vi "DrawAntennas.vi"(8 "Coords":u32[][](array[numeric]), 10 "New Image":T1, 11 "In Image":T1) -> (3 "Out Image":T1)   [LabVIEW 2024]
uses:
  <vilib>/vision/Image Controls.llb/IMAQ Image.ctl
  <vilib>/vision/NI_Vision_Development_Module.lvlib
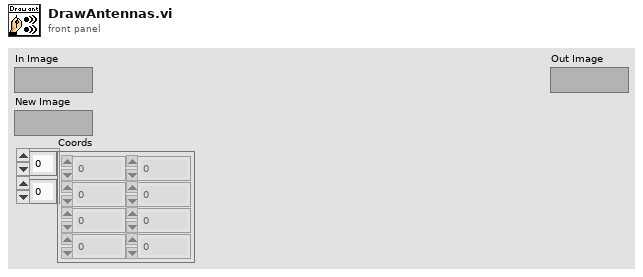
[diagram p1: front panel]
types:
  T1 = typedef "IMAQ Image.ctl" = refnum<image>
  T2 = cluster{"Desired Font (Application)":enum16{"User-specified Font", "Application Font", "System Font", "Dialog Font"}, "[User-specified Font]":cluster{"Font Name":string, "Size":i16, "Strikeout?":bool, "Italic?":bool, "Underline?":bool, "Outline?":bool, "Shadow?":bool, "Bold?":bool, "Rotation Angle":dbl}, "Horizontal Alignment":i16, "Vertical Alignment":i16}
  T3 = cluster{"Red or Hue value":u8, "Green or Sat value":u8, "Blue or Luma or Val or Inten value":u8}
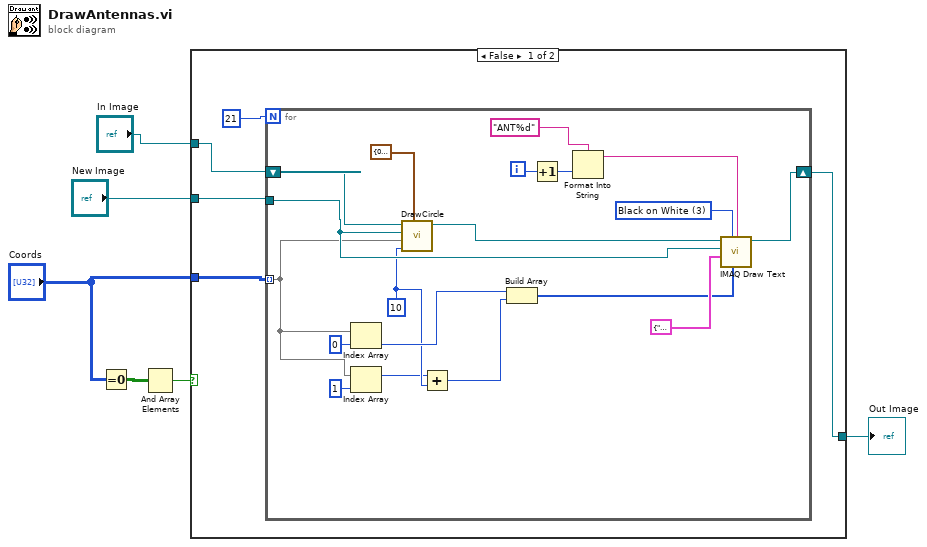
[diagram p0: block diagram]
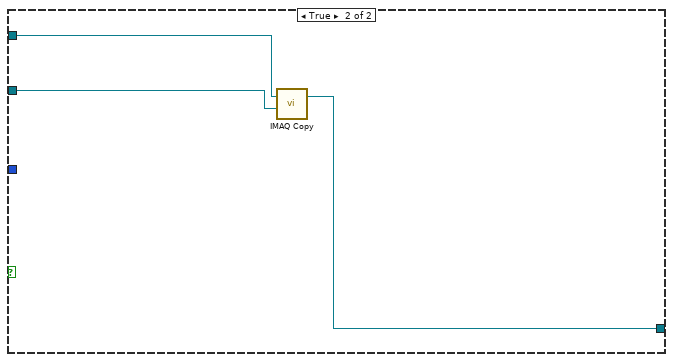
[diagram p2: hidden frame]
diagram:
  n1 = Equal To 0?(x="Coords") -> (x = 0?=w2:bool[][])
  n2 = And Array Elements(Boolean array=w2) -> (logical AND=w1:bool)
  n3 = case shown="False" w1 {
    tunnel: [w10 w31] -> w6
    tunnel: "New Image" -> [w9 w32]
    tunnel: "In Image" -> [w8 w33]
    tunnel: "Coords" -> [w7 _]
    frame False {
      n4 = for {
        N: 21 -> [_]
        tunnel: w7 -> [w17] mode=indexing
        tunnel: w9 -> [w29]
        shift-right: [w27] -> w10
        shift-left: w8 -> [w30]
        i -> [w22]
        w20 = 3 items=["White", "Black", "Inverted", "Black on White", "White on Black"] ("Color")
        w14 = 10 ("Radius")
        n5 = Index Array(array=w17, index=0) -> (element=w16:u32)
        n6 = Index Array(array=w17, index=1) -> (element=w13:u32)
        n7 = call "DrawCircle.vi"("Color"=T3 {"Red or Hue value"=0, "Green or Sat value"=255, "Blue or Luma or Val or Inten value"=0}, "Radius"=w14, "Center coord"=w17, "New Image"=w29, "Refnum in"=w30) -> ("Refnum out"=w28:T1)  [unwired: 6 in]
        n8 = Add(x=w13, y=w14) -> (x+y=w12:u32)
        n9 = Build Array(w16, w12) -> (w15:u32[])
        n10 = Increment(x=w22) -> (x+1=w21:i32)
        n11 = Format Into String(format string="ANT%d" ("String"), w21) -> (resulting string=w23:string)  [unwired: 2 in, 1 out]
        n12 = call "IMAQ Draw Text"("String"=w23, "Insertion Point"=w15, "Color"=w20, "Font, Size & Style"=T2 {"Desired Font (Application)"=enum."User-specified Font", "[User-specified Font]"={"Font Name"="", "Size"=20, "Strikeout?"=FALSE, "Italic?"=FALSE, "Underline?"=FALSE, "Outline?"=FALSE, "Shadow?"=TRUE, "Bold?"=FALSE, "Rotation Angle"=0.0}, "Horizontal Alignment"=1, "Vertical Alignment"=1}, "Image Dst"=w29, "Image Src"=w28) -> ("Image Dst Out"=w27:T1)  [unwired: 2 in, 3 out]
      }
    }
    frame True {
      n13 = call "IMAQ Copy"("Image Dst"=w32, "Image Src"=w33) -> ("Image Dst Out"=w31:T1)  [unwired: 4 in, 1 out]
    }
  }
  "Out Image" <- w6
